vi "3_2.vi"() -> ()   [LabVIEW 2010]
panel:
  out "Array 3":dbl[][][](array[numeric])
  out "Array 2":dbl[][](array[numeric])
  out "Array":dbl[](array[numeric])
  in  "stop":bool
  in  "OK Button":bool
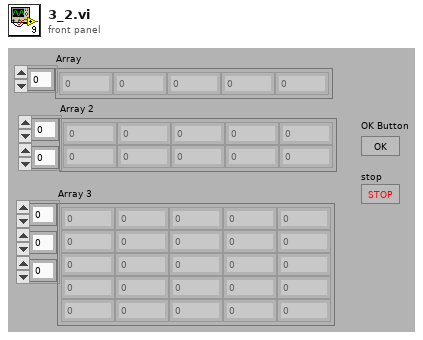
[diagram p1: front panel]
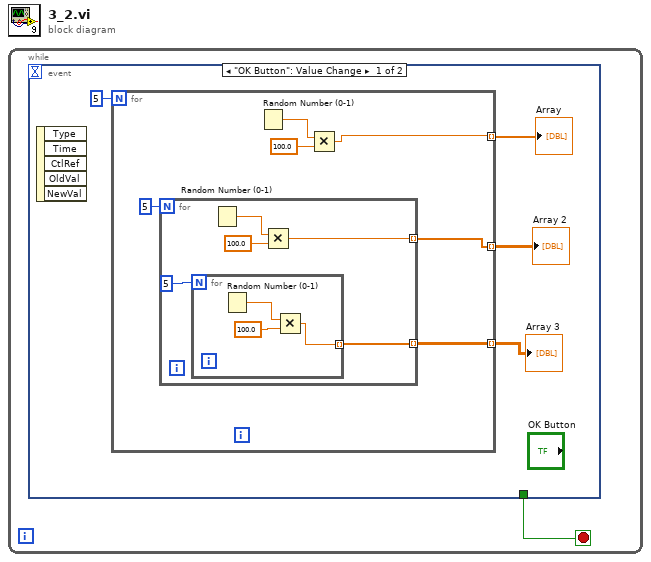
[diagram p0: block diagram]
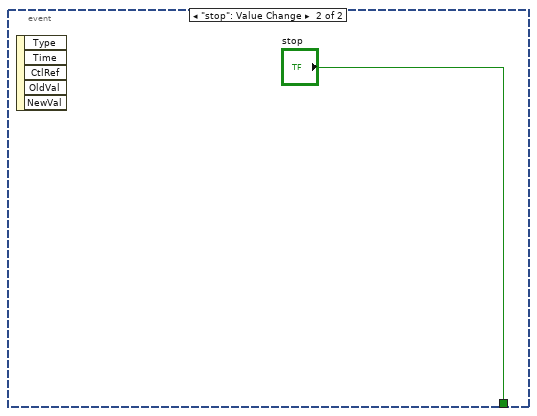
[diagram p2: hidden frame]
diagram:
  n1 = while {
    stop <- w1 stop-if-true
    n2 = event shown="[0] \"OK Button\": Value Change" {
      selector: _ -> [_ _]
      dyn-events: _ -> [_ _]
      timeout: _ -> [_ _]
      tunnel: [_ "stop"] -> w1
      event "OK Button": Value Change {
        n3 = event-data() -> ()  [unwired: 1 in, 5 out]
        n4 = for {
          N: 5 -> [_]
          tunnel: [w11] -> w4 mode=indexing
          tunnel: [w7] -> w3 mode=indexing
          tunnel: [w6] -> w2 mode=indexing
          n5 = for {
            N: 5 -> [_]
            tunnel: [w16] -> w7 mode=indexing
            tunnel: [w12] -> w6 mode=indexing
            n6 = for {
              N: 5 -> [_]
              tunnel: [w19] -> w12 mode=indexing
              n7 = Random Number (0-1)() -> (number: 0 to 1=w18:dbl)
              n8 = Multiply(x=w18, y=100.0) -> (x*y=w19:dbl)
            }
            n9 = Random Number (0-1)() -> (number: 0 to 1=w15:dbl)
            n10 = Multiply(x=w15, y=100.0) -> (x*y=w16:dbl)
          }
          n11 = Random Number (0-1)() -> (number: 0 to 1=w10:dbl)
          n12 = Multiply(x=w10, y=100.0) -> (x*y=w11:dbl)
        }
        "Array" <- w4
        "Array 2" <- w3
        "Array 3" <- w2
      }
      event "stop": Value Change {
        n13 = event-data() -> ()  [unwired: 1 in, 5 out]
      }
    }
  }
